vi "check_empty_SN.vi.vi"(8 "error in (no error)":errorcluster, 11 "SN":string) -> (0 "error out":errorcluster, 2 "Device Type out":T1, 3 "SN ok?":bool)   [LabVIEW 2024]
uses:
  controls/SN_device_type_out.ctl
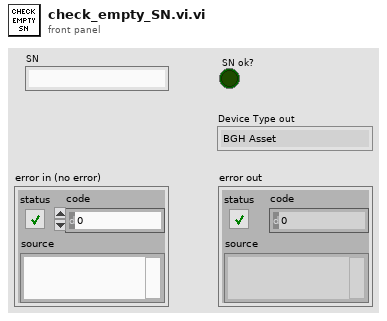
[diagram p1: front panel]
types:
  T1 = typedef "SN_device_type_out.ctl" = enum16{"BGH Asset", "BGH Product", "SAMSUNG Product", "GENERIC Product", "No Product", ""}
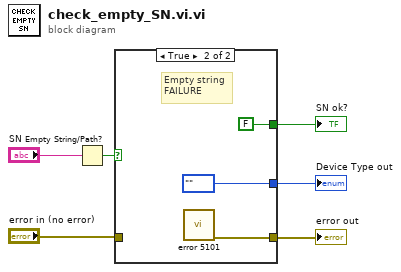
[diagram p0: block diagram]
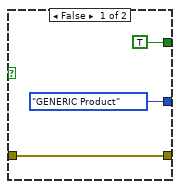
[diagram p2: hidden frame]
diagram:
  n1 = Empty String/Path?(string/path="SN") -> (empty?=w3:bool)
  n2 = case shown="True" w3 {
    tunnel: [TRUE FALSE] -> w1
    tunnel: [w8 w10] -> w6
    tunnel: "error in (no error)" -> [w8 _]
    tunnel: [SN_device_type_out."GENERIC Product" ("Device Type out") SN_device_type_out."" ("Device Type out")] -> w5
    frame False {
    }
    frame True {
      # "Empty string\nFAILURE"
      n3 = call "error 5101.vi"() -> ("error out"=w10:errorcluster)  [unwired: 11 in]
    }
  }
  "error out" <- w6
  "Device Type out" <- w5
  "SN ok?" <- w1
